vi "Pause or Resume VIs.vi"(7 "Tree":refnum<vi>, 8 "error in":errorcluster, 9 "Pause VIs":bool, 10 "VIs":string[](array[string]), 11 "Application in":refnum<vi>) -> (0 "error out":errorcluster)   [LabVIEW 2013, in "LVTM.lvlib"]
uses:
  LVTM.lvlib
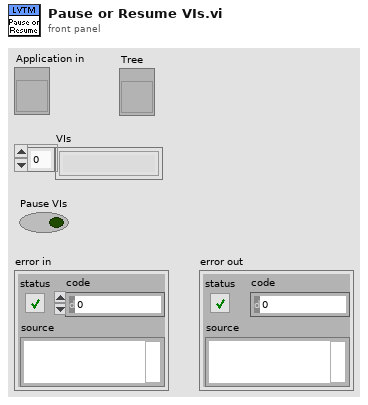
[diagram p1: front panel]
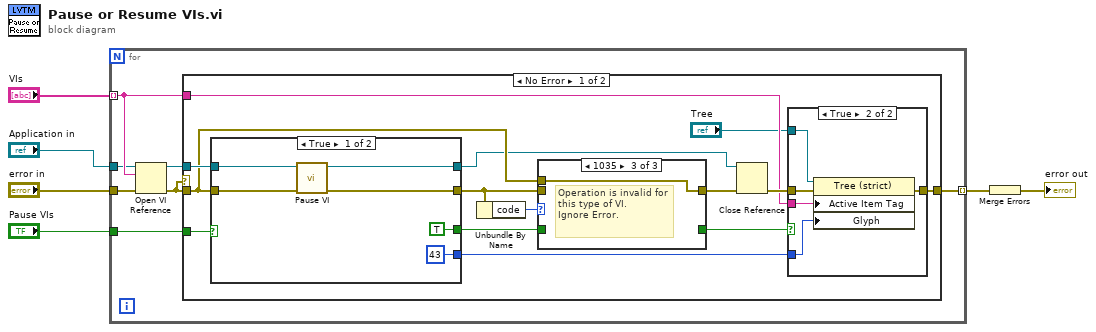
[diagram p0: block diagram]
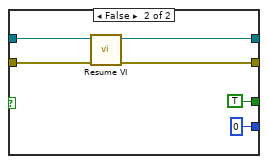
[diagram p5: hidden frame]
diagram:
  n1 = for {
    tunnel: "VIs" -> [w10] mode=indexing
    tunnel: "error in" -> [w12]
    tunnel: [w11] -> w1 mode=indexing
    tunnel: "Application in" -> [w9]
    tunnel: "Pause VIs" -> [w8]
    n2 = Open VI Reference(application reference (local)=w9, vi path=w10, error in (no error)=w12) -> (vi reference=w13:refnum<vi>, error out=w7:errorcluster)  [unwired: 3 out]
    n3 = case shown="No Error" w7 {
      tunnel: w13 -> [w27 _]
      tunnel: [w25 _] -> w11
      tunnel: w10 -> [w24 _]
      tunnel: w7 -> [w19 _]
      tunnel: w8 -> [w17 _]
      frame No Error {
        n4 = case shown="True" w17 {
          tunnel: w19 -> [w43 w49]
          tunnel: w27 -> [w42 w48]
          tunnel: [w41 w46] -> w18
          tunnel: [w40 w47] -> w20
          tunnel: [43 ("Active Item:Symbol Index") 0 ("Active Item:Symbol Index")] -> w23
          tunnel: [TRUE TRUE] -> w15
          frame True {
            n5 = call "Pause VI.vi"("error in (no error)"=w43, "VI in"=w42) -> ("error out"=w40:errorcluster, "VI out"=w41:refnum<vi>)  [unwired: 8 in]
          }
          frame False {
            n6 = call "Resume VI.vi"("error in (no error)"=w49, "VI in"=w48) -> ("error out"=w47:errorcluster, "VI out"=w46:refnum<vi>)  [unwired: 8 in]
          }
        }
        n7 = Unbundle By Name(w20) -> ("code"=w22:i32)
        n8 = case shown="1035" w22 {
          tunnel: [w35 w36 w37] -> w21
          tunnel: w20 -> [w35 w36 _]
          tunnel: w19 -> [_ _ w37]
          tunnel: [w34 _ _] -> w16
          tunnel: w15 -> [w34 _ _]
          frame 0 {
          }
          frame Default {
          }
          frame 1035 {
            # "Operation is invalid for this type of VI.\nIgnore Error."
          }
        }
        n9 = Close Reference(reference=w18, error in (no error)=w21) -> (error out=w26:errorcluster)
        n10 = case shown="True" w16 {
          tunnel: w26 -> [w28 w33]
          tunnel: [w28 w32] -> w25
          tunnel: w24 -> [_ w31]
          tunnel: w23 -> [_ w30]
          tunnel: "Tree" -> [_ w29]
          frame False {
          }
          frame True {
            n11 = property on="Property Node" class="Tree (strict)"(reference=w29, error in=w33, "Active Item Tag"=w31, "Glyph"=w30) -> (error out=w32:errorcluster)  [unwired: 1 out]
          }
        }
      }
      frame Error {
        # "This VI is no longer in the memory"
      }
    }
  }
  n12 = Merge Errors(w1) -> (→"error out":errorcluster)
